vi "UseInvokeNode.vi"   [LabVIEW 2021]
doc: "This VI demonstrates an asynchronous call and forget. When this VI is run, it asynchronously calls a target VI and will not wait for the results. This VI will run to completion while the target VI continues to run.\n\nThis example uses the Start Asynchronous Call method and the Open VI Reference option 0x80.\n\nWhen running this example, notice this VI finishes execution while the target VI continues to run."
panel:
  # "Use Invoke Node"
types:
  T1 = enum32{"Invalid", "Standard", "Closed", "Hidden", "Minimized", "Maximized"}
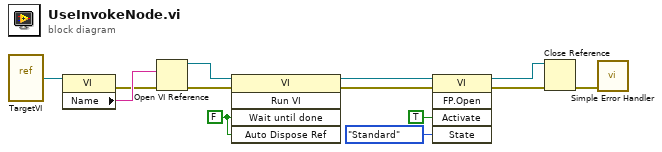
[diagram p0: block diagram]
diagram:
  w6 = FALSE ("Wait Until Done")
  n1 = vi-ref "TargetVI.vi"() -> (w9:refnum<vi>)
  n2 = property class="VI"(reference=w9) -> (error out=w7:errorcluster, "Name"=w8:string)  [unwired: 1 in, 1 out]
  n3 = Open VI Reference(vi path=w8, error in (no error)=w7) -> (vi reference=w13:refnum<vi>, error out=w12:errorcluster)  [unwired: 4 in]
  n4 = invoke class="VI" method="Run VI"(reference=w13, error in=w12, "Wait until done"=w6, "Auto Dispose Ref"=w6) -> (reference out=w4:refnum<vi>, error out=w11:errorcluster)  [unwired: 1 in, 3 out]
  n5 = invoke class="VI" method="FP.Open"(reference=w4, error in=w11, "Activate"=TRUE ("Activate?"), "State"=T1."Standard") -> (reference out=w3:refnum<vi>, error out=w5:errorcluster)  [unwired: 1 in, 3 out]
  n6 = Close Reference(reference=w3, error in (no error)=w5) -> (error out=w10:errorcluster)
  n7 = call <vilib>:"Simple Error Handler.vi"("error in (no error)"=w10) -> ()  [unwired: 4 in, 5 out]
